vi "UtilityLib.unzip.vi"(0 "zipFilePath":path, 1 "targetDirectory":path, 5 "error in (no error)":errorcluster, 7 "previewOnly":bool) -> (14 "dup zipFilePath":path, 15 "Unzipped files":path[](array[path]), 19 "error out":errorcluster)   [LabVIEW 2014, in "UtilityLib.lvlib"]
doc: "Extracts a zip file"
uses:
  UtilityLib.lvlib
  <vilib>/zip/NI_Unzip.lvlib
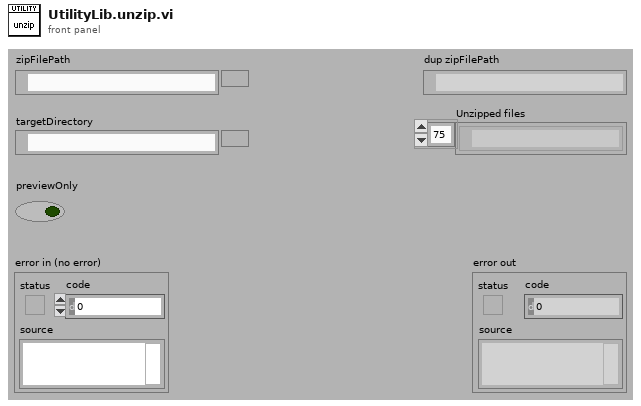
[diagram p1: front panel]
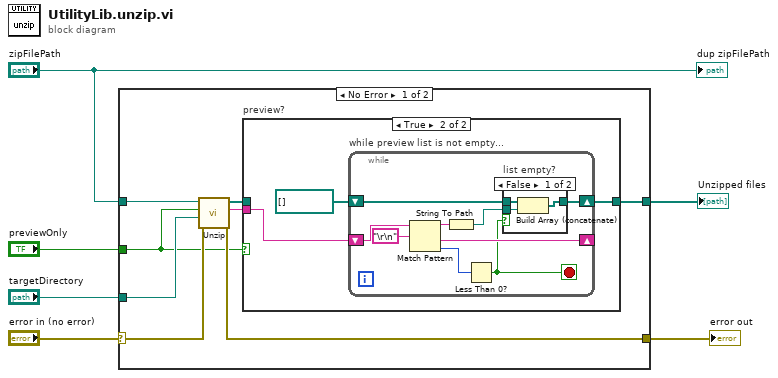
[diagram p0: block diagram]
diagram:
  n1 = case shown="No Error" "error in (no error)" {
    selector: "error in (no error)" -> [w11 w32]
    tunnel: "previewOnly" -> [w10 _]
    tunnel: "targetDirectory" -> [w14 _]
    tunnel: [w13 w32] -> w4
    tunnel: "zipFilePath" -> [w12 _]
    tunnel: [w8 _] -> w1
    frame No Error {
      n2 = call <vilib>:"Unzip.vi"("error in (no error)"=w11, "Target directory (same as Zip file if empty)"=w14, "Preview only?"=w10, "Zip file"=w12) -> ("error out"=w13:errorcluster, "Preview"=w7:string, "Unzipped files"=w9:path[])  [unwired: 5 in]
      n3 = case "preview?" shown="True" w10 {
        tunnel: w9 -> [w15 _]
        tunnel: [w15 w16] -> w8
        tunnel: w7 -> [_ w17]
        frame False {
        }
        frame True {
          n4 = while "while preview list is not empty..." {
            shift-right: [w21] -> w16
            shift-left: path[] [] -> [w24]
            shift-right: [w20] -> _
            shift-left: w17 -> [w26]
            stop <- w19 stop-if-true
            n5 = Match Pattern(string=w26, regular expression="\r\n") -> (before substring=w23:string, after substring=w20:string, offset past match=w25:i32)  [unwired: 1 in, 1 out]
            n6 = String To Path(string=w23) -> (path=w22:path)
            n7 = Less Than 0?(x=w25) -> (x < 0?=w19:bool)
            n8 = case "list empty?" shown="False" w19 {
              tunnel: w24 -> [w30 w31]
              tunnel: w22 -> [w29 _]
              tunnel: [w28 w31] -> w21
              frame False {
                n9 = Build Array (concatenate)(w30, w29) -> (w28:path[])
              }
              frame True {
              }
            }
          }
        }
      }
    }
    frame Error {
    }
  }
  "error out" <- w4
  "Unzipped files" <- w1
  "dup zipFilePath" <- "zipFilePath"
